vi "Test Skipped.vi"(11 "Test Case In":refnum<class "Skipped Test.lvclass">) -> (0 "error out":errorcluster, 3 "Test Case Out":refnum<class "Skipped Test.lvclass">)   [LabVIEW 2020, in "Skipped Test.lvclass"]
uses:
  Skipped Test.lvclass
  C:/git/astemes-lunit/source/LUnit Test Case.lvclass
  source/LUnit Test Case.lvclass/LUnit Test Case.ctl
  source/LUnit Test Case.lvclass
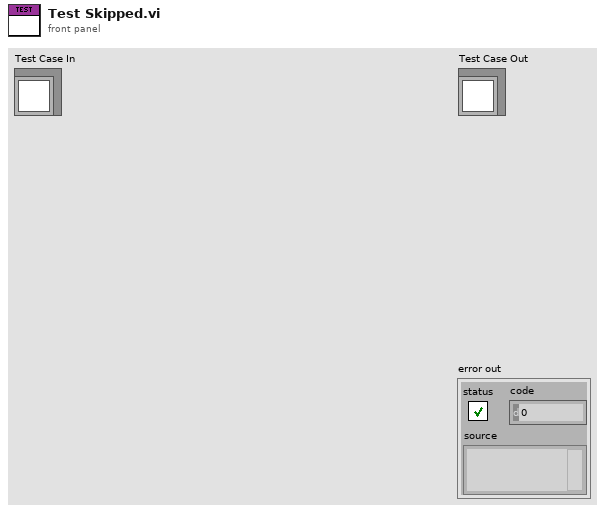
[diagram p1: front panel]
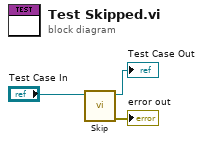
[diagram p0: block diagram]
diagram:
  n1 = call "Skip.vi"("LUnit Test Case In"="Test Case In") -> ("error out"=→"error out":errorcluster, "LUnit Test Case Out"=→"Test Case Out":refnum<class "Skipped Test.lvclass">)  [unwired: 9 in]
